vi "Actor Core.vi"(8 "error in":errorcluster, 11 "Measure Object in":refnum<class "Line Detector.lvclass">) -> (0 "error out":errorcluster, 3 "Actor out":refnum<class "Actor.lvclass">)   [LabVIEW 2016, in "Line Detector.lvclass"]
doc: "Line Detector module finds amplitude peaks in spectrum file and fits complex Lorentzian around peaks"
uses:
  Line Detector.lvclass
  C:/github/LabActor/Template Module/Template Module.lvclass
  C:/Program Files (x86)/National Instruments/LabVIEW 2016/vi.lib/ActorFramework/Actor/Actor.lvclass
  <vilib>/ActorFramework/Actor/Actor.lvclass
  Line Detector Configuration.ctl
  Line Detector.lvclass/Line Detector.ctl
  Template Module/Template Module.lvclass/Template Module.ctl
  <vilib>/ActorFramework/Actor/Actor.lvclass/Actor.ctl
  <vilib>/ActorFramework/Message Enqueuer/Message Enqueuer.lvclass/Message Enqueuer.ctl
  Results/File Path Result/File Path Result.lvclass
  C:/github/LabActor/Results/Acquired Result/Acquired Result.lvclass
  Process Object Messages/Process Result Msg/Process Result Msg.lvclass/Process Result Msg.ctl
  Template Module/Read stop event.vi
  <vilib>/ActorFramework/Message Enqueuer/Init from Existing Queue.vi
  <vilib>/ActorFramework/Message Enqueuer/Enqueue.vi
  Process Object Messages/Process Result Msg/Process Result Msg.lvclass
  C:/Program Files (x86)/National Instruments/LabVIEW 2016/vi.lib/ActorFramework/Message/Message.lvclass
  <vilib>/ActorFramework/Message Priority Queue/Priority Enqueue.vi
  Process Object/Process Object.lvclass
  <vilib>/ActorFramework/Message Enqueuer/Message Enqueuer.lvclass
panel:
  in  "Best fit results":dbl[][](array[numeric]) format="%#_10p"
  in  "Plot Tab Control":enum32{"Spectrum fit", "Peak finder"}(tab)
  out "Spectrum fit":cluster{dbl[], dbl[]}[](graph)
  out "Peak Plot":cluster{"Ramp Pattern":dbl[], "X":dbl[]}[](graph)
  out "Name":string
  in  "Re-process":bool
  in  "Configuration":T1={"Peak width guess"=500.0, "Background removal"=enum."High-pass", "Smoothing"=enum."Low-pass", "Smooth window"=200.0, "Relative threshold"=0.2, "Finder algorithm"=enum."Wavelet", "Bgd window"=50000.0, "Spectrum recorder module name"="Spectrum Recorder", "Fit window"=1000.0, "Initial fit guess"=enum."Peak finder", "...with header "="test\n2 0 12 0 1.3396 1.00 1 0 0 0 0 0 0 0 0 0\n0.5 0.16\n.5 .2", "Follow\npeaks"=FALSE, "Re-sample"=nan, "rusin\n.dat"=enum."NONE"} {"Re-sample" format="%#_6pHz"; "Fit window" format="%#_6pHz"; "Bgd window" format="%#_6pHz"; "Smooth window" format="%#_6pHz"; "Peak width guess" format="%#_6pHz"}
  in  "Input file":path
  # "f0     |     g     |    A    |   q    |    Xbg   |  Ybg"
  # "Peak finder config"
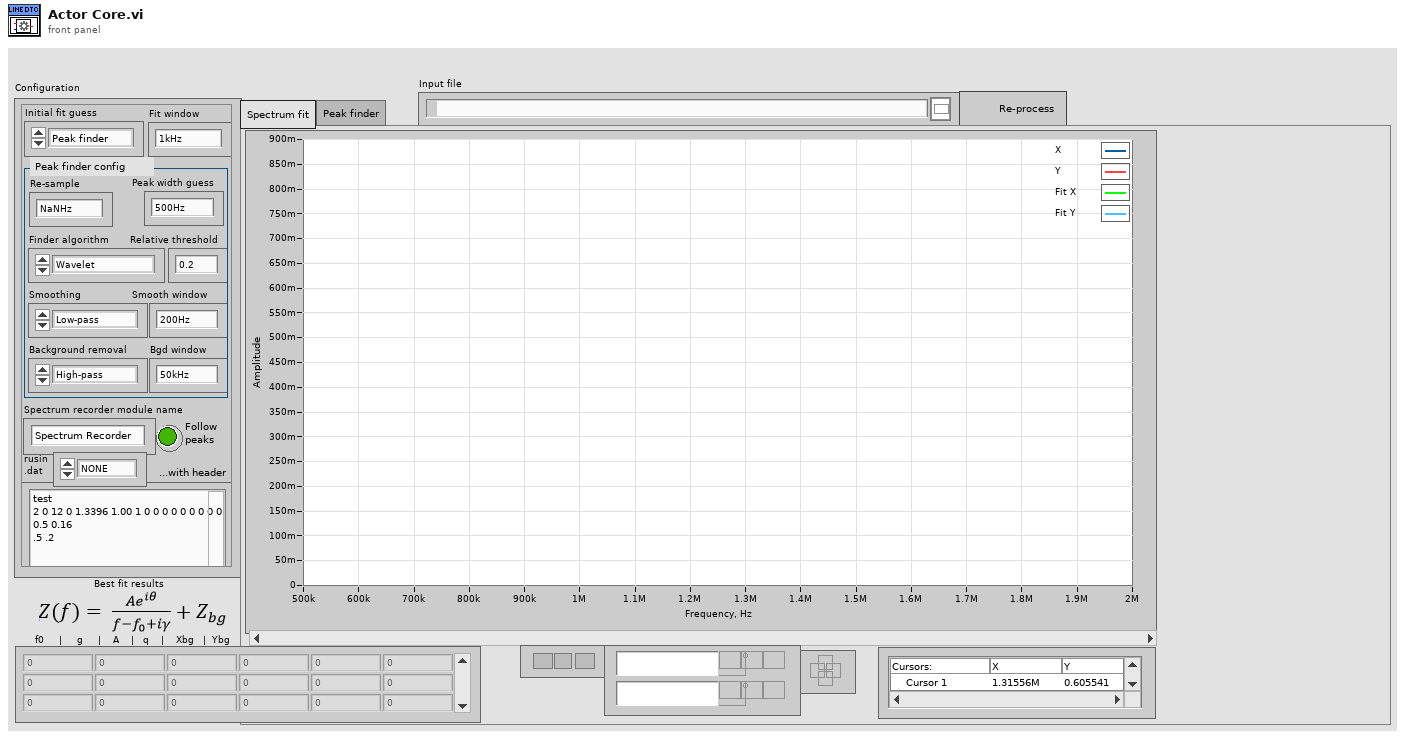
[diagram p1: front panel]
types:
  T1 = typedef "Line Detector Configuration.ctl" = cluster{"Peak width guess":dbl, "Background removal":enum16{"NONE", "High-pass", "Detrend"}, "Smoothing":enum16{"NONE", "Low-pass", "Denoise"}, "Smooth window":dbl, "Relative threshold":dbl, "Finder algorithm":enum16{"Basic", "Wavelet", "Wavelet+detrend"}, "Bgd window":dbl, "Spectrum recorder module name":string, "Fit window":dbl, "Initial fit guess":enum16{"Peak finder", "Last fit"}, "...with header ":string, "Follow\npeaks":bool, "Re-sample":dbl, "rusin\n.dat":enum16{"NONE", "DINES/cm2", "GPa"}}
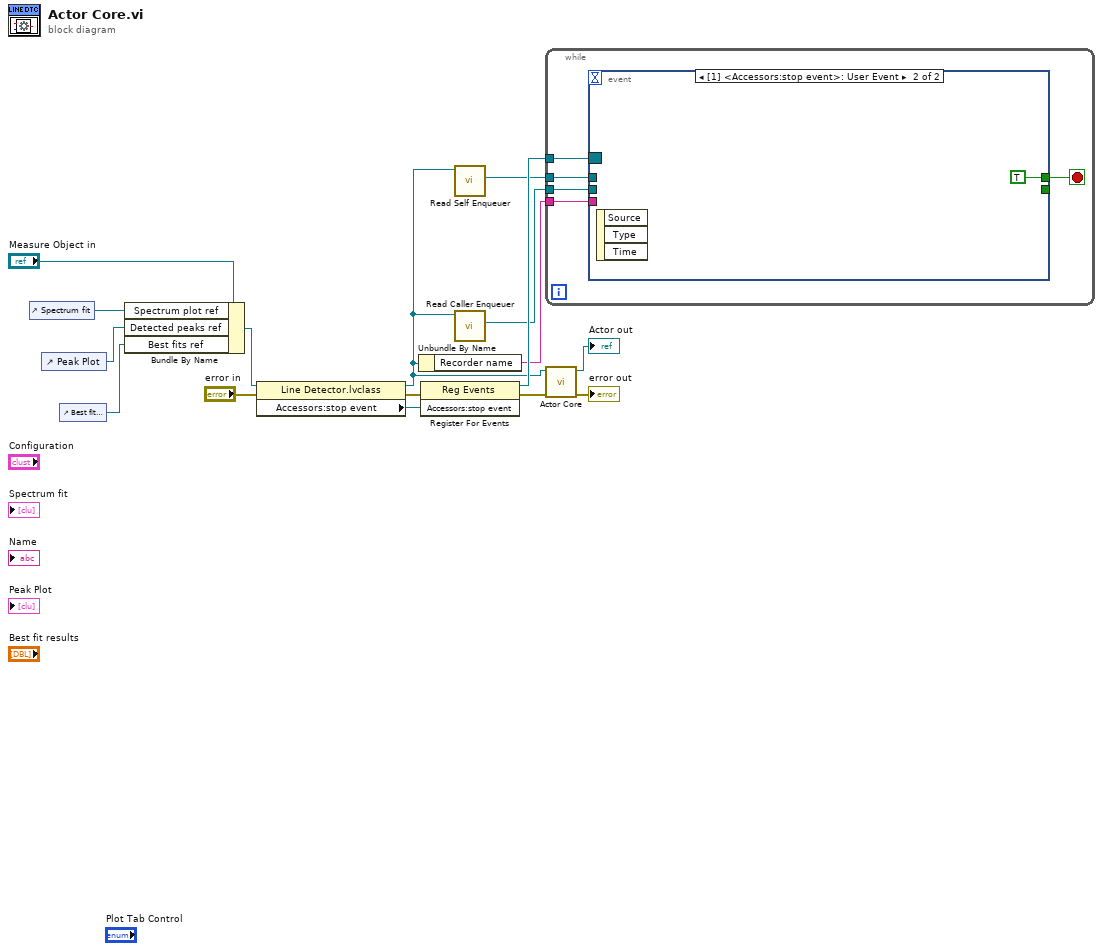
[diagram p0: block diagram]
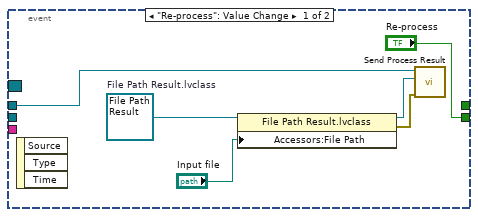
[diagram p2: hidden frame]
diagram:
  n1 = control-ref of="Spectrum fit"() -> (w7:refnum<vi>)
  n2 = control-ref of="Peak Plot"() -> (w6:refnum<vi>)
  n3 = control-ref of="Best fit results"() -> (w5:refnum<vi>)
  n4 = Bundle By Name(cluster="Measure Object in", "Spectrum plot ref"=w7, "Detected peaks ref"=w6, "Best fits ref"=w5) -> (w8:refnum<class "Line Detector.lvclass">)
  n5 = property class="Line Detector.lvclass"(reference=w8, error in="error in") -> (reference out=w2:refnum<class "Line Detector.lvclass">, error out=w12:errorcluster, "Accessors:stop event"=w14:refnum<user-event>)
  n6 = Unbundle By Name(w2) -> ("Recorder name"=w1:string)
  n7 = register-events(error in=w12, w14) -> (reference out=w13:refnum<event-registration>, error out=w4:errorcluster)  [unwired: 1 in]
  n8 = call <vilib>:"Read Self Enqueuer.vi"("Actor"=w2) -> ("Self Enqueuer"=w11:refnum<class "Message Enqueuer.lvclass">)  [unwired: 10 in]
  n9 = call <vilib>:"Read Caller Enqueuer.vi"("Actor"=w2) -> ("Caller Enqueuer"=w3:refnum<class "Message Enqueuer.lvclass">)  [unwired: 10 in]
  n10 = while {
    tunnel: w13 -> [w21]
    tunnel: w11 -> [w19]
    tunnel: w3 -> [w18]
    tunnel: w1 -> [w17]
    stop <- w20 stop-if-true
    n11 = event shown="[1] <Accessors:stop event>: User Event" {
      selector: w21 -> [_ _]
      dyn-events: _ -> [_ _]
      timeout: _ -> [_ _]
      tunnel: [_ TRUE] -> w20
      tunnel: w19 -> [w27 _]
      tunnel: ["Re-process" _] -> _
      tunnel: w18 -> [_ _]
      tunnel: w17 -> [_ _]
      event "Re-process": Value Change {
        w26 = refnum<class "File Path Result.lvclass"> refnum  # File Path Result.lvclass
        n12 = event-data() -> ()  [unwired: 1 in, 3 out]
        n13 = property class="File Path Result.lvclass"(reference=w26, "Accessors:File Path"="Input file") -> (reference out=w25:refnum<class "File Path Result.lvclass">, error out=w24:errorcluster)  [unwired: 1 in]
        n14 = call "Send Process Result.vi"("error in (no error)"=w24, "Result in"=w25, "Message Enqueuer"=w27) -> ()  [unwired: 7 in, 2 out]
      }
      event User Event {
        n15 = event-data() -> ()  [unwired: 1 in, 3 out]
      }
    }
  }
  n16 = call-parent "Actor Core.vi"("error in"=w4, "Measure Object in"=w2) -> ("error out"=→"error out":errorcluster, "Actor out"=→"Actor out":refnum<class "Actor.lvclass">)  [unwired: 8 in]
